vi "publishConnected.vi"(8 "error in (no error)":errorcluster, 10 "Connected":bool=TRUE, 11 "TCPCommunicator in":refnum<class "TCPCommunicator.lvclass">) -> (0 "error out":errorcluster, 3 "TCPCommunicator out":refnum<class "TCPCommunicator.lvclass">)   [LabVIEW 2016, in "TCPCommunicator.lvclass"]
uses:
  TCPCommunicator.lvclass
  TCPCommunicator.lvclass/TCPCommunicator.ctl
  TCPComEvents/TCPComEvents.lvclass
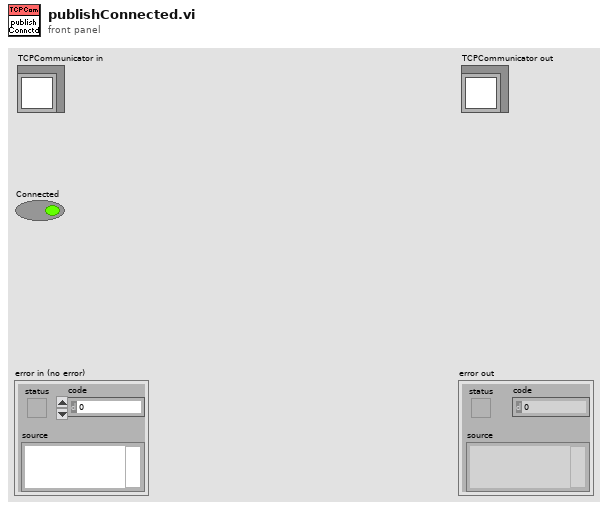
[diagram p1: front panel]
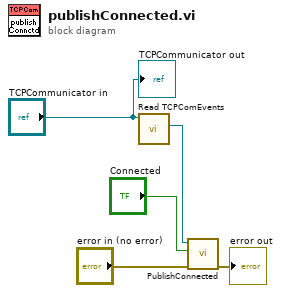
[diagram p0: block diagram]
diagram:
  n1 = call "Read TCPComEvents.vi"("TCPCommunicator in"="TCPCommunicator in") -> ("TCPComEvents.lvclass"=w2:refnum<class "TCPComEvents.lvclass">)  [unwired: 8 in, 2 out]
  n2 = call "PublishConnected.vi"("error in (no error)"="error in (no error)", "Connected"="Connected", "TCPComEvents in"=w2) -> ("error out"=→"error out":errorcluster)  [unwired: 7 in, 1 out]
  "TCPCommunicator out" <- "TCPCommunicator in"
